vi "get boards in chain.vi"(8 "error in (no error)":errorcluster, 10 "devs":u16, 11 "identifier":string) -> (0 "error out":errorcluster, 2 "devs out":u16, 3 "function return":bool)   [LabVIEW 2015, in "XGL_DPP.lvlib"]
doc: "EXTERN DECLSPEC bool CALL_CONV get_boards_in_chain(const char * identifier, uint16_t * devs);"
uses:
  XGL_DPP.lvlib
  XGL_DPP.dll
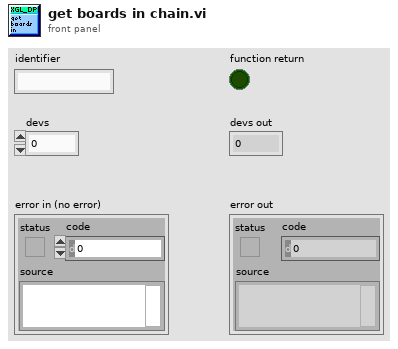
[diagram p1: front panel]
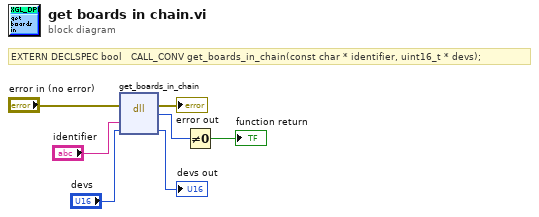
[diagram p0: block diagram]
diagram:
  # "EXTERN DECLSPEC bool   CALL_CONV get_boards_in_chain(const char * identifier, uint16_t * devs);"
  n1 = dll-call lib="D:/Users/XRF/Desktop/Scanning Software_Demokritos_2015_v7/libs/Vis_2/XGL_DPP.*" fn="get_boards_in_chain"(error in="error in (no error)", "identifier"="identifier", "devs"="devs") -> (error out=→"error out":errorcluster, w6:u8, "devs"=→"devs out":u16)  [unwired: 3 in, 1 out]
  n2 = Not Equal To 0?(x=w6) -> (x != 0?=→"function return":bool)
